vi "Set Timeout.vi"(8 "error in (no error)":errorcluster, 10 "Timeout":i32, 11 "SwipeMenu in":refnum<class "SwipeMenu.lvclass">) -> (0 "error out":errorcluster, 3 "SwipeMenu out":refnum<class "SwipeMenu.lvclass">)   [LabVIEW 2019, in "SwipeMenu.lvclass"]
uses:
  SwipeMenu.lvclass
  SwipeMenu.lvclass/SwipeMenu.ctl
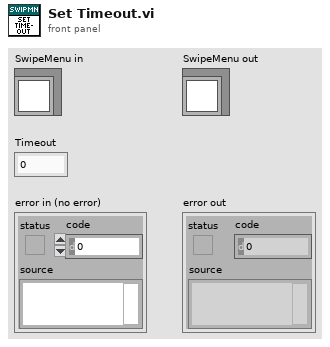
[diagram p1: front panel]
types:
  T1 = typedef "SwipeMenu.lvclass/State Data.ctl" = cluster{"State":enum16{"Idle", "Mouse Nav", "Slowdown", "Button Nav"}, "Timeout":i32, "Time":timestamp, "Position":i32, "Scroll Position":i16, "Rate":dbl, "Direction":enum16{"Left", "Right"}}
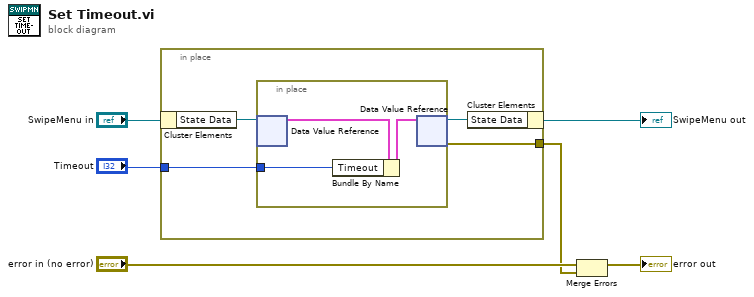
[diagram p0: block diagram]
diagram:
  n1 = in-place {
    in-place-border: [w8] -> w2
    in-place-border: "Timeout" -> [w7]
    n2 = in-place-cluster #1("SwipeMenu in") -> ("State Data"=w10:refnum<data-value>)
    n3 = in-place {
      in-place-border: w7 -> [w11]
      n4 = in-place-dvr #2(w10) -> (w13:T1)  [unwired: 1 out]
      n5 = Bundle By Name(cluster=w13, "Timeout"=w11) -> (w12:T1)
      n6 = in-place-dvr #2(w12) -> (w9:refnum<data-value>, w8:errorcluster)
    }
    n7 = in-place-cluster #1("State Data"=w9) -> (→"SwipeMenu out":refnum<class "SwipeMenu.lvclass">)
  }
  n8 = Merge Errors("error in (no error)", w2) -> (→"error out":errorcluster)
